vi "test Add Connections.vi"(8 "error in (no error)":errorcluster, 11 "TestCase in":refnum<class "Switch Scripting Unit Tests.lvclass">) -> (0 "error out":errorcluster, 3 "TestCase out":refnum<class "Switch Scripting Unit Tests.lvclass">)   [LabVIEW 2017, in "Switch Scripting Unit Tests.lvclass"]
uses:
  Switch Scripting Unit Tests.lvclass
  Shared/Routing State.ctl
  Shared/Connection.ctl
  Switch Scripting Unit Tests.lvclass/Switch Scripting Unit Tests.ctl
  <vilib>/addons/_JKI Toolkits/VI Tester/TestCase.llb/TestCase.lvclass
  Switch Scripting.lvlib
  Shared/Routing and Faulting Shared.lvlib
  C:/Program Files (x86)/National Instruments/LabVIEW 2017/vi.lib/addons/_JKI Toolkits/VI Tester/TestCase.llb/TestCase.lvclass
panel:
  in  "Save?":bool
  out "Output Filename":string
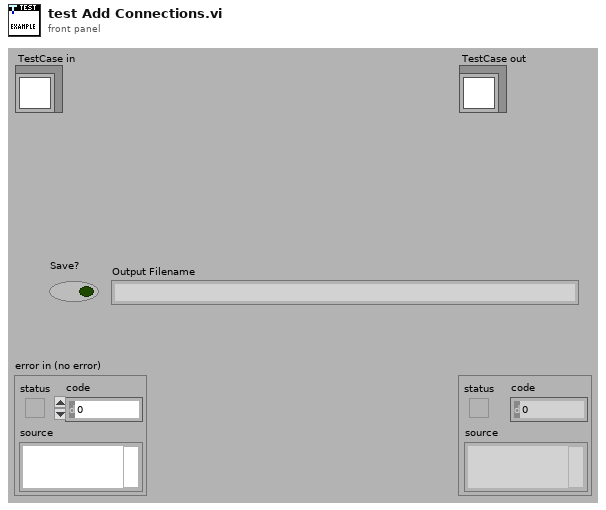
[diagram p1: front panel]
types:
  T1 = typedef "Routing and Faulting Shared.lvlib/Connection.ctl" = cluster{"Source":string, "Destination":string}
  T2 = typedef "Routing and Faulting Shared.lvlib/Routing State.ctl" = cluster{"Name":string, "Description":string, "Value":i32, "Connection List":T1[]}
  T3 = typedef "Custom Device API.lvlib/Custom Device Item Ref.ctl" = u64
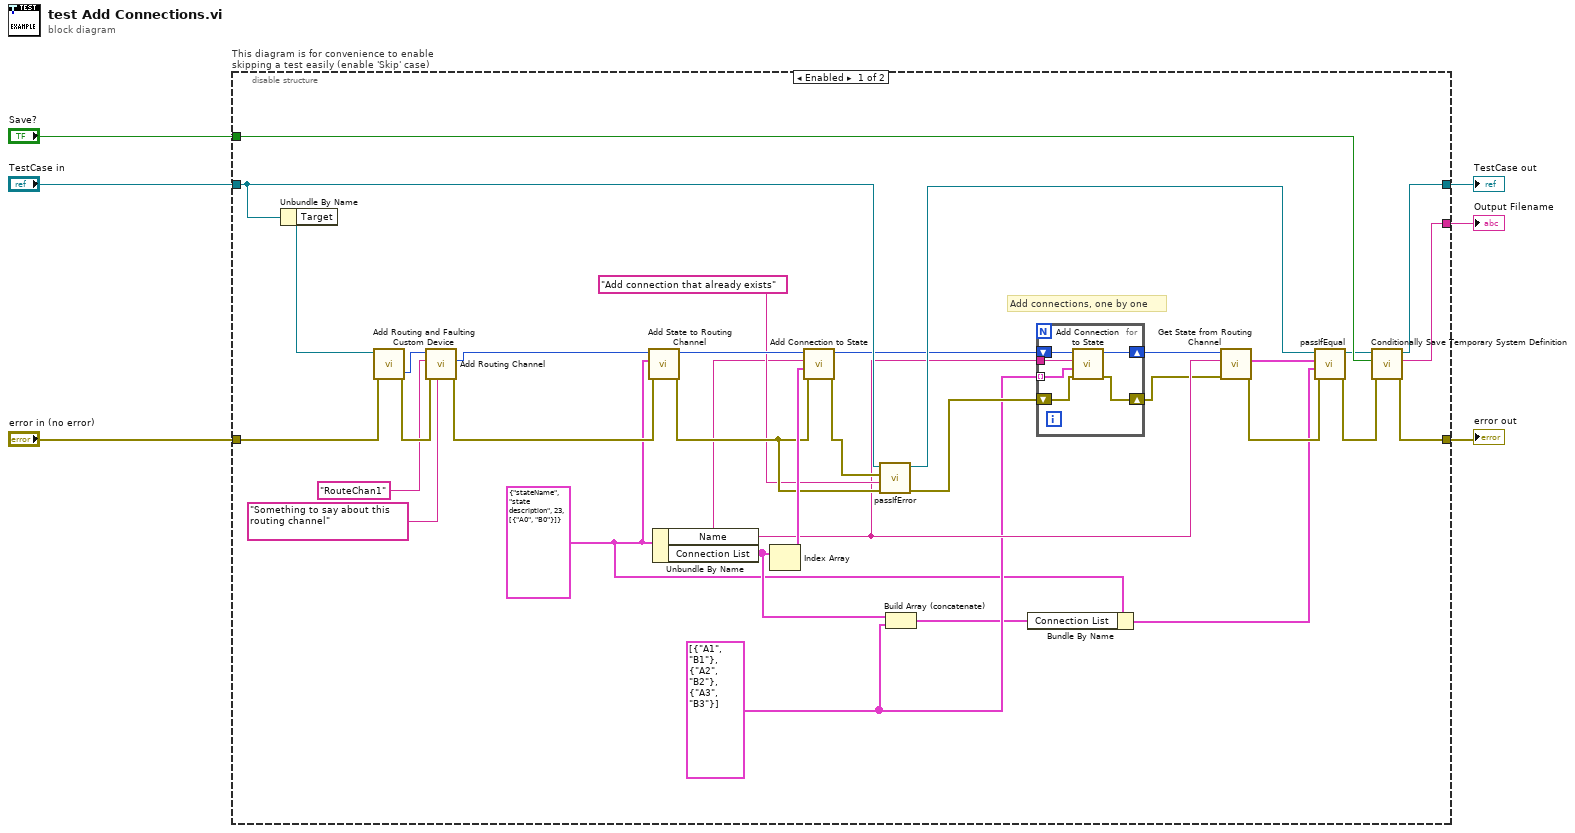
[diagram p0: block diagram]
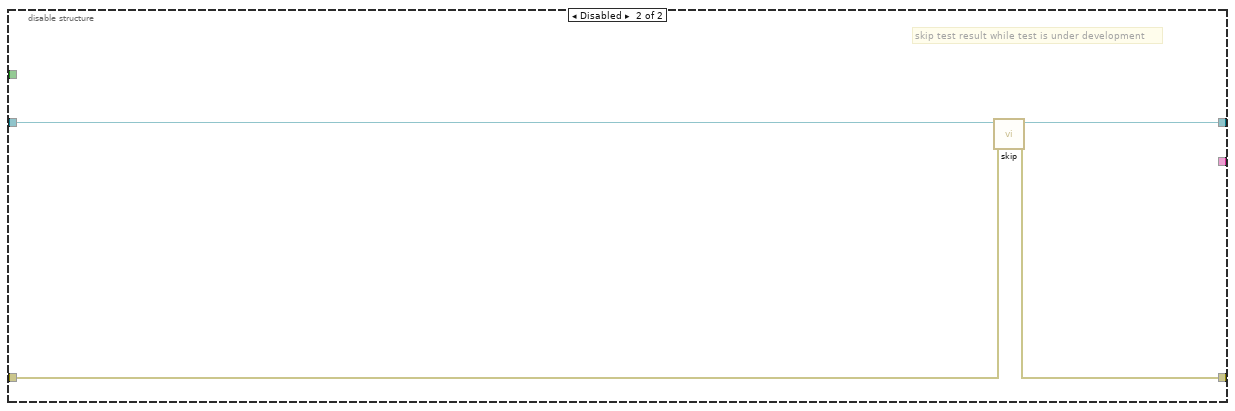
[diagram p2: hidden frame]
diagram:
  n1 = disable-structure "This diagram is for convenience to enable skipping a test easily (enable 'Skip' case)" shown="Enabled" {
    disable-tunnel: "TestCase in" -> [w22 w49]
    disable-tunnel: [w34 w47] -> w3
    disable-tunnel: [w38 w48] -> w5
    disable-tunnel: "error in (no error)" -> [w39 w46]
    disable-tunnel: [w37 _] -> w2
    disable-tunnel: "Save?" -> [w36 _]
    frame Enabled {
      w10 = T1[] [{"Source"="A1", "Destination"="B1"}, {"Source"="A2", "Destination"="B2"}, {"Source"="A3", "Destination"="B3"}] ("connection list")
      w9 = T2 {"Name"="stateName", "Description"="state description", "Value"=23, "Connection List"=[{"Source"="A0", "Destination"="B0"}]} ("Routing State")
      # "Add connections, one by one"
      n2 = Unbundle By Name(w22) -> ("Target"=w35:refnum<k24>)
      n3 = call "Add Routing and Faulting Custom Device.vi"("error in (no error)"=w39, "Target in"=w35) -> ("error out"=w33:errorcluster, "Routes Section Ref"=w30:T3)  [unwired: 5 in, 3 out]
      n4 = call "Add Routing Channel.vi"("Description"="Something to say about this routing channel", "error in (no error)"=w33, "Channel Name"="RouteChan1", "Routes Ref in"=w30) -> ("error out"=w25:errorcluster, "Channel Ref"=w24:T3)  [unwired: 5 in, 1 out]
      n5 = call "Add State to Routing Channel.vi"("error in (no error)"=w25, "Routing State"=w9, "Channel Ref in"=w24) -> ("error out"=w18:errorcluster, "Channel Ref out"=w23:T3)  [unwired: 7 in]
      n6 = Unbundle By Name(w9) -> ("Name"=w16:string, "Connection List"=w11:T1[])
      n7 = Index Array(array=w11) -> (element=w20:T1)  [unwired: 1 in]
      n8 = call "Add Connection to State.vi"("error in (no error)"=w18, "Connection"=w20, "State"=w16, "Channel Ref in"=w23) -> ("error out"=w19:errorcluster, "Channel Ref out"=w14:T3)  [unwired: 6 in]
      n9 = call-dynamic "passIfError.vi"("error in (no error)"=w18, "task (\"\")"="Add connection that already exists" ("task (\"\")"), "error"=w19, "TestCase in"=w22) -> ("error out"=w15:errorcluster, "TestCase out"=w21:refnum<class "Switch Scripting Unit Tests.lvclass">)  [unwired: 6 in]
      n10 = Build Array (concatenate)(w11, w10) -> (w8:T1[])
      n11 = Bundle By Name(cluster=w9, "Connection List"=w8) -> (w7:T2)
      n12 = for {
        tunnel: w16 -> [w45]
        tunnel: w10 -> [w44] mode=indexing
        shift-right: [w40] -> w12
        shift-left: w15 -> [w43]
        shift-right: [w42] -> w13
        shift-left: w14 -> [w41]
        n13 = call "Add Connection to State.vi"("error in (no error)"=w43, "Connection"=w44, "State"=w45, "Channel Ref in"=w41) -> ("error out"=w40:errorcluster, "Channel Ref out"=w42:T3)  [unwired: 6 in]
      }
      n14 = call "Get State from Routing Channel.vi"("error in (no error)"=w12, "State"=w16, "Channel Ref in"=w13) -> ("error out"=w29:errorcluster, "Routing State"=w28:T2)  [unwired: 6 in, 1 out]
      n15 = call-dynamic "passIfEqual.vi"("error in (no error)"=w29, "y"=w7, "x"=w28, "TestCase in"=w21) -> ("error out"=w32:errorcluster, "TestCase out"=w31:refnum<class "Switch Scripting Unit Tests.lvclass">)  [unwired: 6 in]
      n16 = call "Conditionally Save Temporary System Definition.vi"("error in (no error)"=w32, "Save?"=w36, "Test Case"=w31) -> ("error out"=w38:errorcluster, "filename"=w37:string, "Test Case"=w34:refnum<class "Switch Scripting Unit Tests.lvclass">)  [unwired: 6 in]
    }
    frame Disabled {
      # "skip test result while test is under development"
      n17 = call <vilib>:"skip.vi"("error in (no error)"=w46, "TestCase in"=w49) -> ("error out"=w48:errorcluster, "TestCase out"=w47:refnum<class "Switch Scripting Unit Tests.lvclass">)  [unwired: 8 in]
    }
  }
  "error out" <- w5
  "TestCase out" <- w3
  "Output Filename" <- w2
